vi "Get Page VI.vi"(8 "error in (no error)":errorcluster, 9 "GUID":string, 10 "Item Ref":T1 format="%.0x", 11 "System Explorer Dispatcher Implementation in":refnum<class "System Explorer Dispatcher.lvclass">) -> (0 "error out":errorcluster, 2 "page reference":refnum<vi>, 3 "System Explorer Dispatcher Implementation out":refnum<class "System Explorer Dispatcher.lvclass">)   [LabVIEW 2020, in "AIM ARINC 429 System Explorer.lvlib" / "Implementation.lvlib" / "System Explorer Dispatcher.lvclass"]
uses:
  System Explorer Dispatcher.lvclass
  <vilib>/NI VeriStand/Custom Device API/Custom Device Item Ref.ctl
  Scripting/AIM/Constants.vi
  Implementation.lvlib
  Scripting/AIM/AIM ARINC 429 Scripting.lvlib
  <vilib>/NI VeriStand/Custom Device API/Custom Device API.lvlib
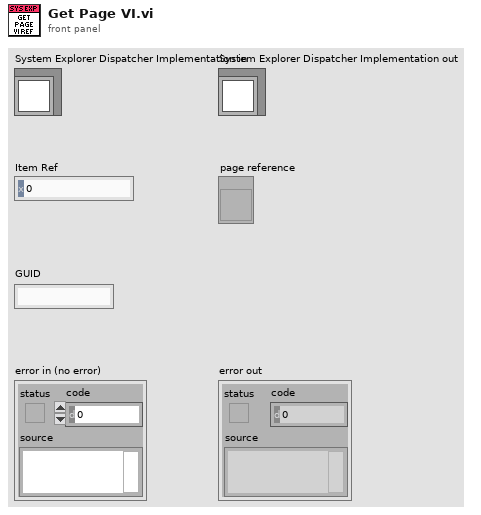
[diagram p1: front panel]
types:
  T1 = typedef "Custom Device API.lvlib/Custom Device Item Ref.ctl" = u64
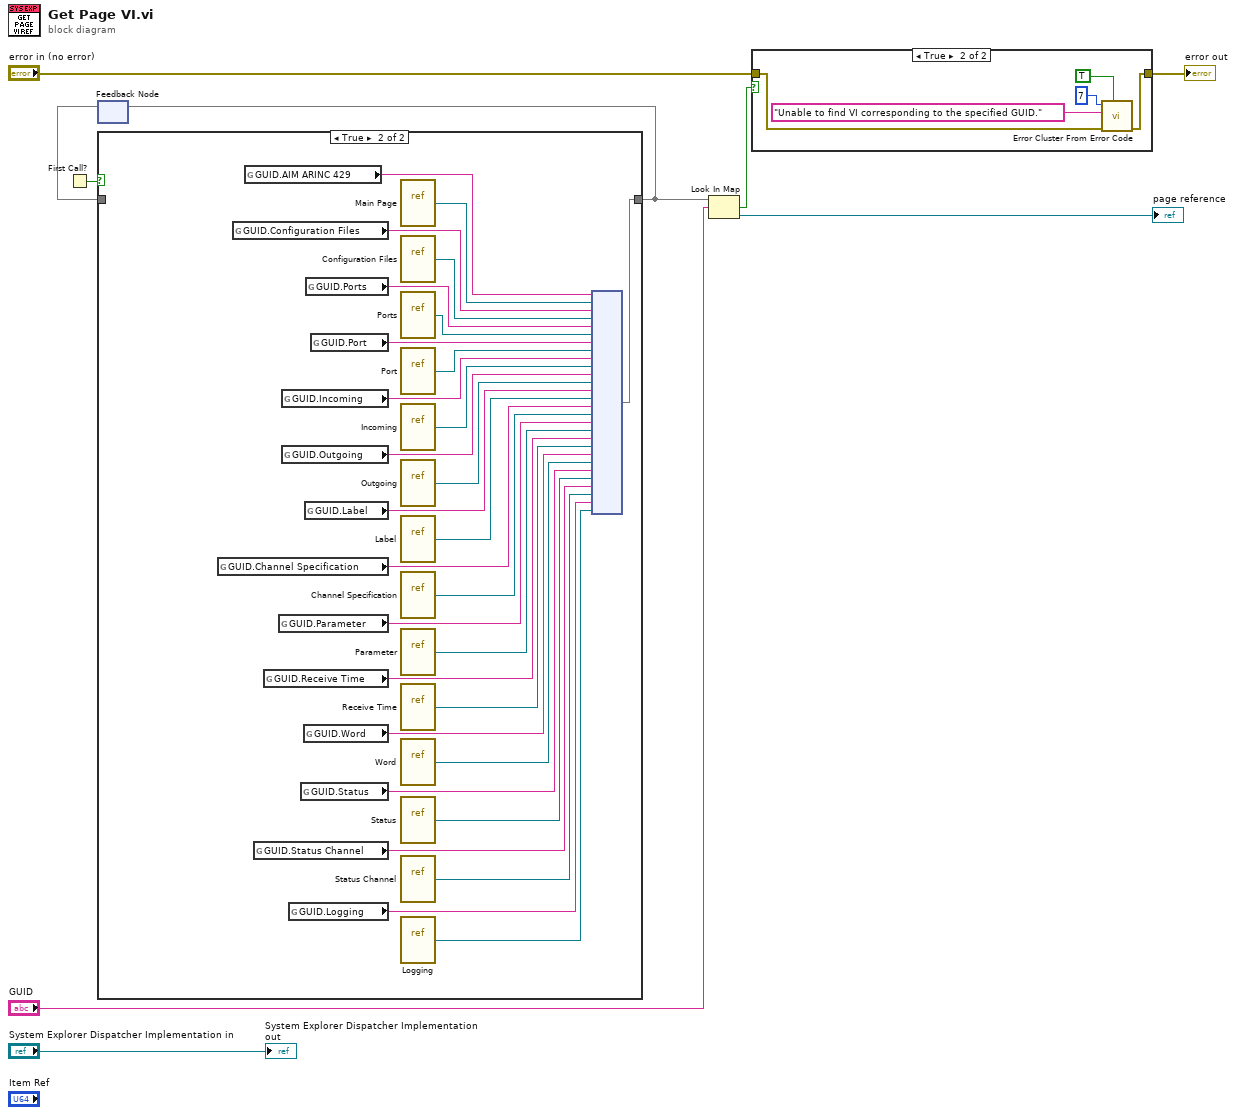
[diagram p0: block diagram]
diagram:
  n1 = First Call?() -> (First Call?: T/F=w8:bool)
  n2 = feedback #1() -> (w7:map{string, refnum<vi>})  [unwired: 1 in]
  n3 = case shown="True" w8 {
    tunnel: [w10 w39] -> w6
    tunnel: w7 -> [w10 _]
    frame False {
    }
    frame True {
      n4 = global read "Constants.vi" "GUID.Channel Specification"() -> (w24:string)
      n5 = global read "Constants.vi" "GUID.Configuration Files"() -> (w35:string)
      n6 = global read "Constants.vi" "GUID.AIM ARINC 429"() -> (w37:string)
      n7 = global read "Constants.vi" "GUID.Status Channel"() -> (w14:string)
      n8 = global read "Constants.vi" "GUID.Receive Time"() -> (w20:string)
      n9 = global read "Constants.vi" "GUID.Parameter"() -> (w22:string)
      n10 = global read "Constants.vi" "GUID.Incoming"() -> (w30:string)
      n11 = global read "Constants.vi" "GUID.Outgoing"() -> (w28:string)
      n12 = global read "Constants.vi" "GUID.Logging"() -> (w12:string)
      n13 = global read "Constants.vi" "GUID.Status"() -> (w16:string)
      n14 = global read "Constants.vi" "GUID.Word"() -> (w18:string)
      n15 = global read "Constants.vi" "GUID.Label"() -> (w26:string)
      n16 = global read "Constants.vi" "GUID.Ports"() -> (w34:string)
      n17 = global read "Constants.vi" "GUID.Port"() -> (w32:string)
      n18 = vi-ref "Main Page.vi"() -> (w38:refnum<vi>)
      n19 = vi-ref "Configuration Files.vi"() -> (w36:refnum<vi>)
      n20 = vi-ref "Ports.vi"() -> (w33:refnum<vi>)
      n21 = vi-ref "Port.vi"() -> (w31:refnum<vi>)
      n22 = vi-ref "Incoming.vi"() -> (w29:refnum<vi>)
      n23 = vi-ref "Outgoing.vi"() -> (w27:refnum<vi>)
      n24 = vi-ref "Label.vi"() -> (w25:refnum<vi>)
      n25 = vi-ref "Channel Specification.vi"() -> (w23:refnum<vi>)
      n26 = vi-ref "Parameter.vi"() -> (w21:refnum<vi>)
      n27 = vi-ref "Receive Time.vi"() -> (w19:refnum<vi>)
      n28 = vi-ref "Word.vi"() -> (w17:refnum<vi>)
      n29 = vi-ref "Status.vi"() -> (w15:refnum<vi>)
      n30 = vi-ref "Status Channel.vi"() -> (w13:refnum<vi>)
      n31 = vi-ref "Logging.vi"() -> (w11:refnum<vi>)
      n32 = node(w37, w38, w35, w36, w34, w33, w32, w31, w30, w29, w28, w27, w26, w25, w24, w23, w22, w21, w20, w19, w18, w17, w16, w15, w14, w13, w12, w11) -> (w39:map{string, refnum<vi>})
    }
  }
  n33 = feedback-in #1(w6) -> ()
  n34 = Look In Map(map=w6, key="GUID") -> (key not found?=w4:bool, value=→"page reference":refnum<vi>)  [unwired: 1 in]
  n35 = case shown="True" w4 {
    tunnel: [w40 w42] -> w3
    tunnel: "error in (no error)" -> [w40 w41]
    frame False {
    }
    frame True {
      n36 = call <vilib>:"Error Cluster From Error Code.vi"("show call chain? (False)"=TRUE, "error in (no error)"=w41, "error message (\"\")"="Unable to find VI corresponding to the specified GUID." ("error message (\"\")"), "error code (0)"=7) -> ("error out"=w42:errorcluster)  [unwired: 5 in]
    }
  }
  "error out" <- w3
  "System Explorer Dispatcher Implementation out" <- "System Explorer Dispatcher Implementation in"
